vi "水样测试.vi"(11 "数据标记表":string(combo)="N") -> ()   [LabVIEW 2016, in "斯坦道多参数.lvlib"]
panel:
  out "运行状态":u16(ring) items=["空闲", "水样测试", "标样核查"]
  out "多参数运行日志":string
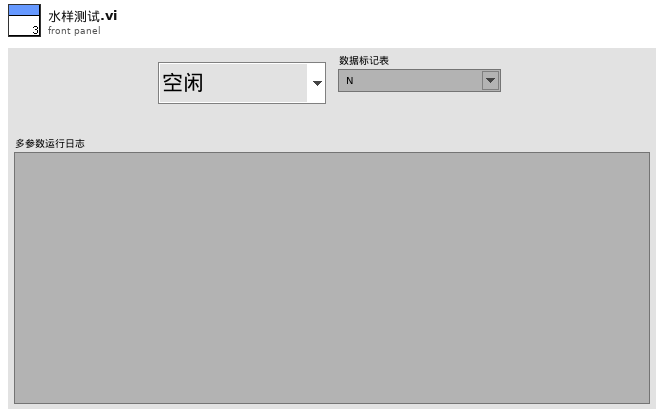
[diagram p1: front panel]
types:
  T1 = typedef "集成多参数单参数字段定义.ctl" = cluster{"时间":timestamp, "测量模式":string, "数据类型":string, "检测值":sgl, "单位":string, "数据标识":string, "标样参考值":sgl, "因子编码":string, "LastTime":timestamp}
  T2 = cluster{"水温":bool, "pH":bool, "DO":bool, "DOper":bool, "电导率":bool, "ORP":bool, "浊度":bool, "叶绿素a":bool, "藻密度":bool, "COD":bool, "DO2":bool, "DOper":bool, "氯化物":bool, "氨氮":bool, "水中油":bool}
  T3 = cluster{"ph":bool, "DO":bool, "Cond":bool, "Turb":bool, "叶绿素a":bool, "藻密度":bool, "ORP":bool, "cod":bool, "DO2":bool, "氯化物":bool, "氨氮":bool, "水中油":bool}
  T4 = cluster{"温度测量值":sgl, "测量值":sgl, "温度偏移修正值":sgl, "信号值":sgl, "数据标识":string}
  T5 = cluster{"温度测量值":sgl, "DO%":sgl, "DOmg/L":sgl, "温度偏移修正值":sgl, "数据标识mg/L":string, "数据标识%":string}
  T6 = cluster{"CH":u16, "监测值":dbl, "信号值":sgl, "数据标识":string}
  T7 = cluster{"水样数据时间":timestamp, "水温":dbl, "pH":dbl, "DO":dbl, "DOper":dbl, "电导率":dbl, "ORP":dbl, "浊度":dbl, "叶绿素a":dbl, "藻密度":dbl, "COD":dbl, "DO2":dbl, "DO2per":dbl, "氯化物":dbl, "氨氮":dbl, "水中油":dbl}
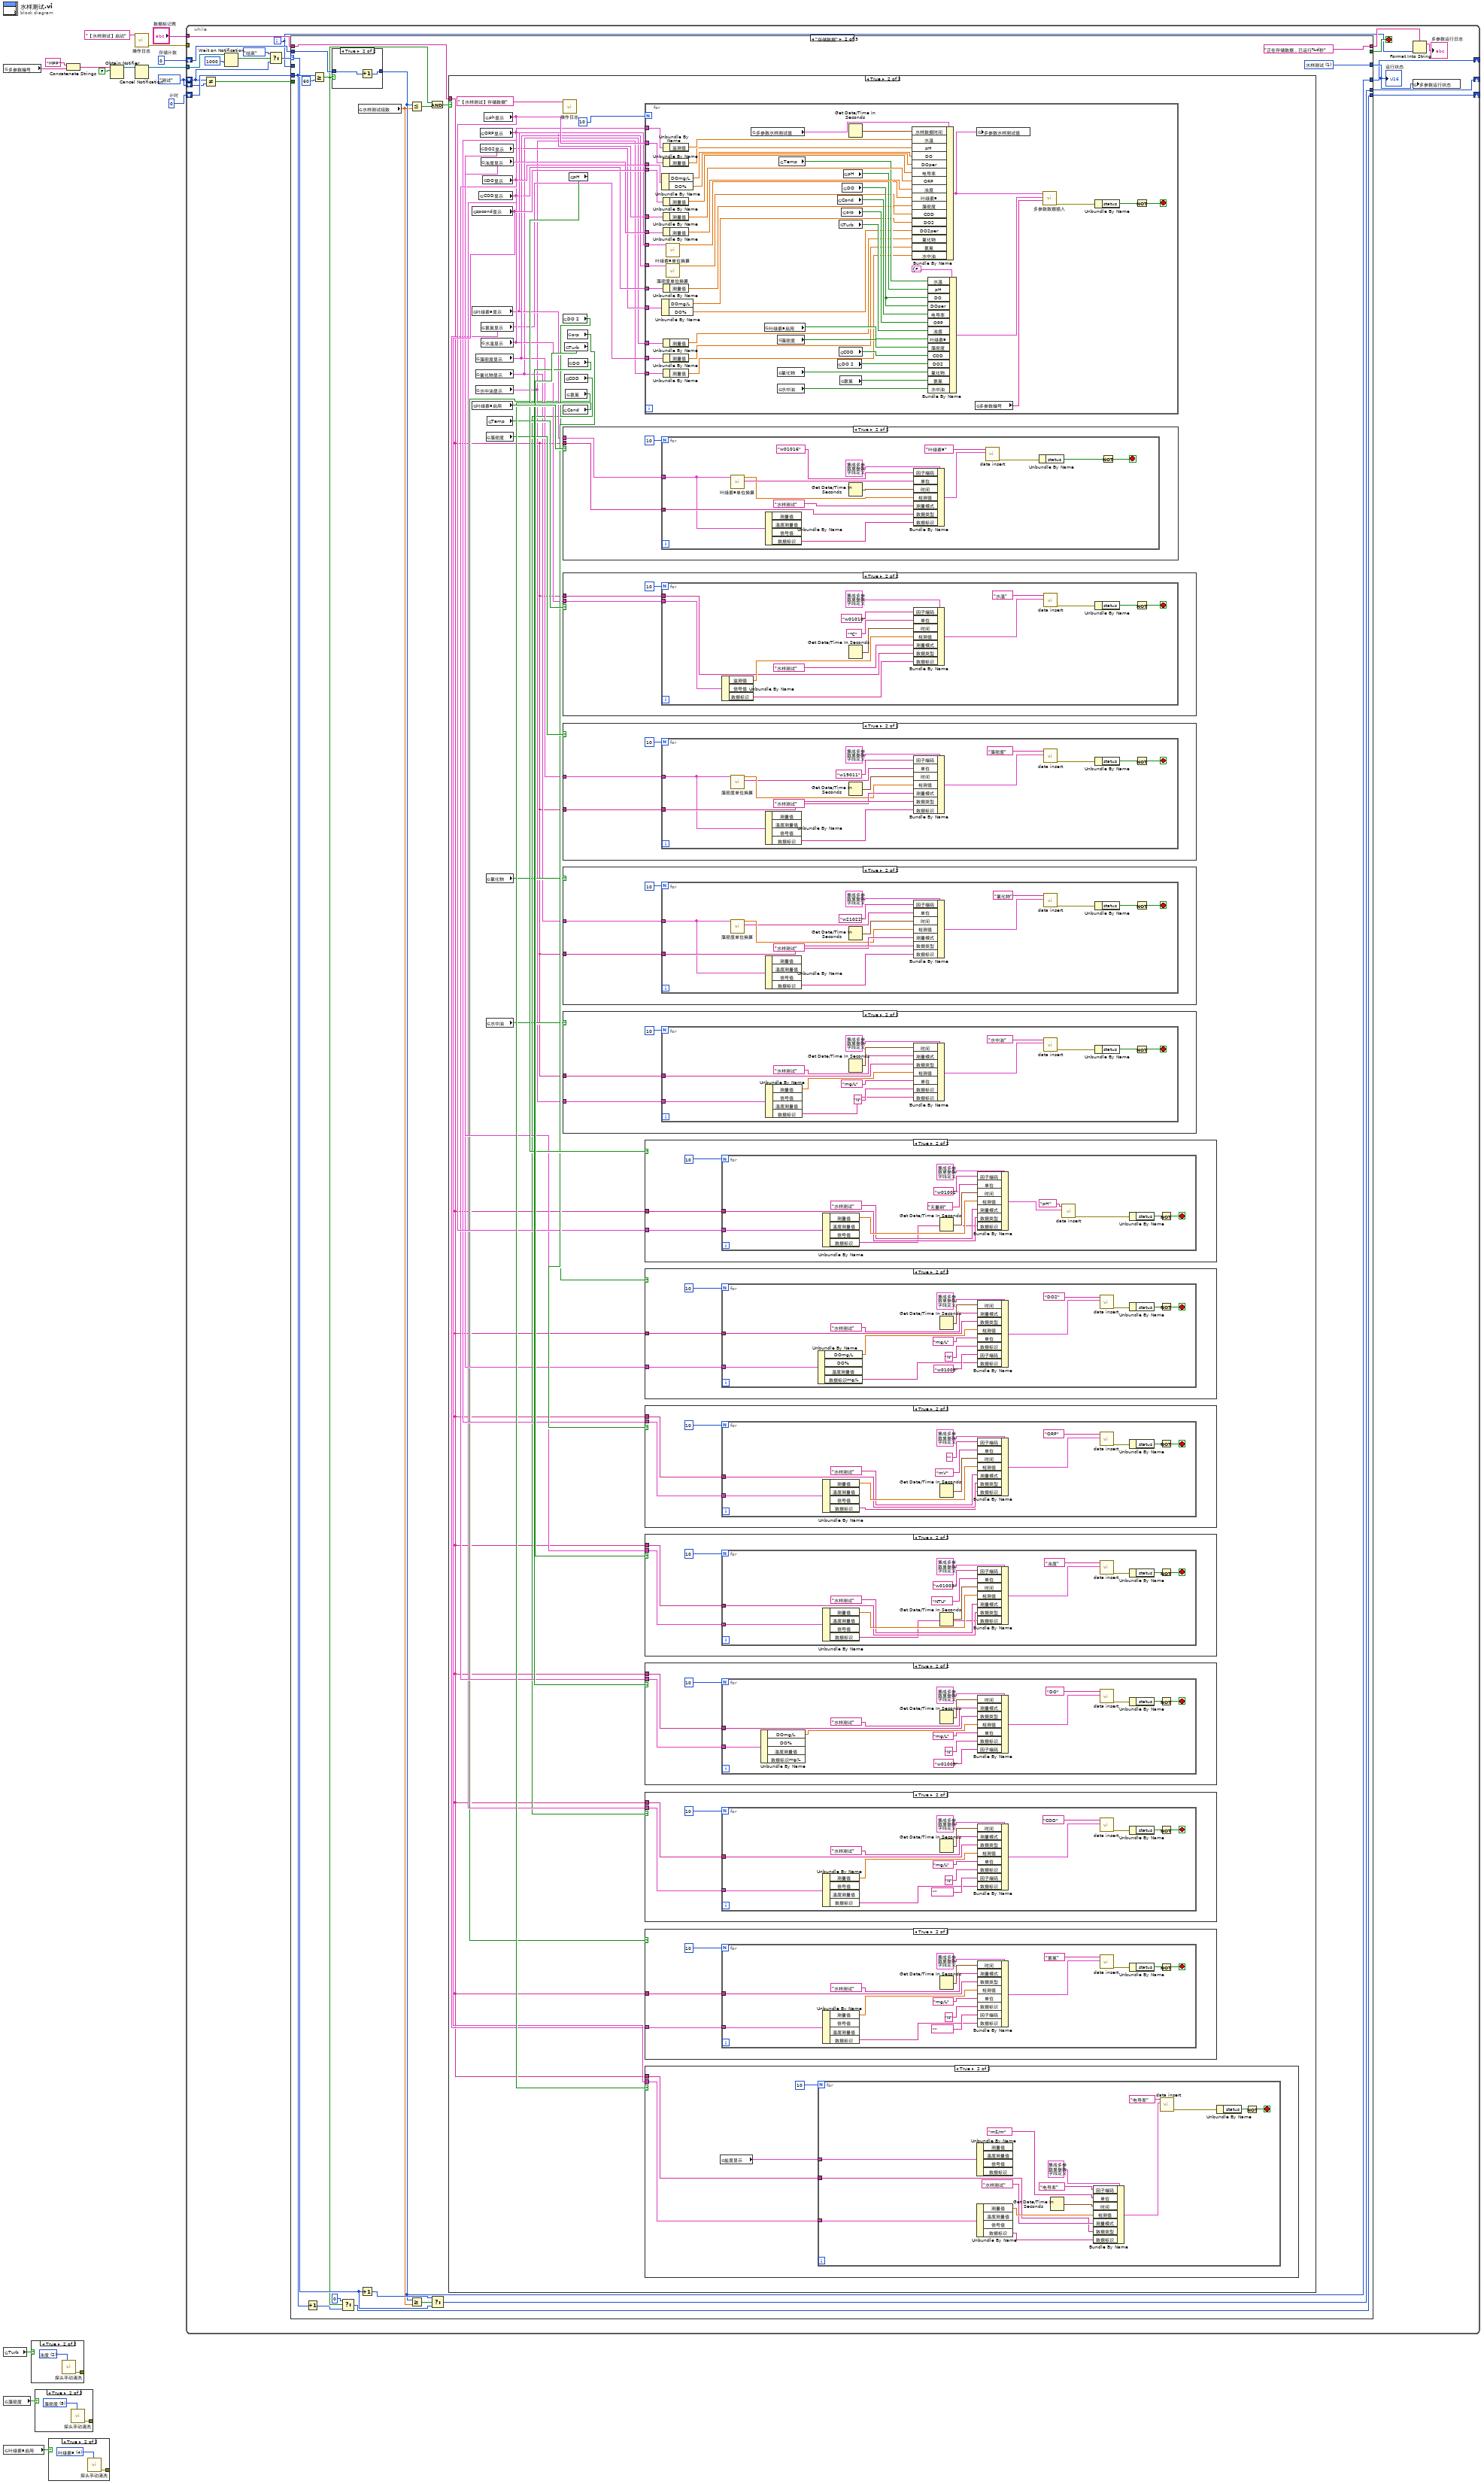
[diagram p0: block diagram]
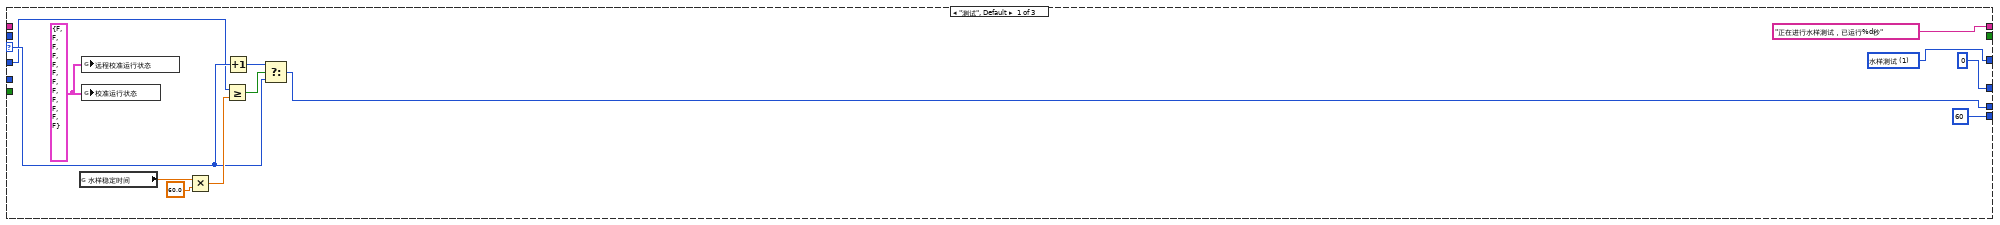
[diagram p5: hidden frame]
diagram:
  w7 = 0  # 存储计数
  w8 = 0  # 计时
  w3 = enum16{"测试", "存储数据", "结束"}."测试" ("枚举")
  n1 = global read "多参数全局变量.vi" "多参数编号"() -> (w9:string)
  n2 = global read "断电保存变量.vi" "Turb"() -> (w6:bool)
  n3 = global read "断电保存变量.vi" "藻密度"() -> (w4:bool)
  n4 = global read "断电保存变量.vi" "叶绿素a启用"() -> (w5:bool)
  n5 = case shown="True" w6 {
    tunnel: [_ w16] -> _
    frame False {
    }
    frame True {
      w17 = u16 2 items=["pH", "DO", "浊度", "电导率", "叶绿素a", "藻密度", "ORP", "DO2"] ("校准参数")
      n6 = call "探头手动清洗.vi"("校准参数"=w17) -> ("error out"=w16:errorcluster)  [unwired: 10 in]
    }
  }
  n7 = case shown="True" w4 {
    tunnel: [_ w18] -> _
    frame False {
    }
    frame True {
      w19 = u16 5 items=["pH", "DO", "浊度", "电导率", "叶绿素a", "藻密度", "ORP", "DO2"] ("校准参数")
      n8 = call "探头手动清洗.vi"("校准参数"=w19) -> ("error out"=w18:errorcluster)  [unwired: 10 in]
    }
  }
  n9 = case shown="True" w5 {
    tunnel: [_ w20] -> _
    frame False {
    }
    frame True {
      w21 = u16 4 items=["pH", "DO", "浊度", "电导率", "叶绿素a", "藻密度", "ORP", "DO2"] ("校准参数")
      n10 = call "探头手动清洗.vi"("校准参数"=w21) -> ("error out"=w20:errorcluster)  [unwired: 10 in]
    }
  }
  n11 = Concatenate Strings("MPP" ("名称（未命名）"), w9) -> (w10:string)
  n12 = Obtain Notifier(name (unnamed)=w10, notification data type=FALSE) -> (notifier out=w13:refnum<notifier>)  [unwired: 2 in, 2 out]
  n13 = call "操作日志.vi"("日志信息"="【水样测试】启动") -> ("error out"=w1:errorcluster)  [unwired: 10 in]
  n14 = Cancel Notification(0:w13) -> (8:w12:refnum<notifier>)  [unwired: 1 in, 2 out]
  n15 = while {
    shift-right: [w26] -> _
    shift-left: w3 -> [w24]
    tunnel: w12 -> [w37]
    tunnel: "数据标记表" -> [w32]
    shift-right: [w28] -> _
    shift-left: w8 -> [w30]
    shift-right: [w27] -> _
    shift-left: w7 -> [w29]
    shift-left: w3 -> [w23]
    tunnel: w1 -> [_]
    i -> [w25]
    stop <- w40 stop-if-true
    n16 = Not Equal?(x=w24, y=w23) -> (x != y?=w22:bool)
    n17 = Wait on Notification(notifier=w37, timeout in ms (-1)=1000 ("超时毫秒(-1)")) -> (notification=w35:bool)  [unwired: 2 in, 3 out]
    n18 = Select(t=enum16{"测试", "存储数据", "结束"}."结束" ("枚举"), s=w35, f=w24) -> (s? t:f=w33:enum16{"测试", "存储数据", "结束"})
    n19 = case shown="\"存储数据\"" w33 {
      selector: w33 -> [w47 w61 _]
      tunnel: [_ _ TRUE] -> w40
      tunnel: ["正在进行水样测试，已运行%d秒" ("格式字符串") "正在存储数据，已运行%d秒" ("格式字符串") "测试停止，累计运行%d秒" ("格式字符串")] -> w39
      tunnel: [w52 w66 w384] -> w31
      tunnel: w32 -> [_ w71 _]
      tunnel: w30 -> [_ w69 _]
      tunnel: w29 -> [_ w70 _]
      tunnel: [60 w54 0] -> w28
      tunnel: [0 w60 0] -> w27
      tunnel: [w45 w64 enum16{"测试", "存储数据", "结束"}."结束" ("枚举")] -> w26
      tunnel: w25 -> [w42 _ _]
      tunnel: w22 -> [_ _ w380]
      frame "测试", Default {
        w41 = T3 {"ph"=FALSE, "DO"=FALSE, "Cond"=FALSE, "Turb"=FALSE, "叶绿素a"=FALSE, "藻密度"=FALSE, "ORP"=FALSE, "cod"=FALSE, "DO2"=FALSE, "氯化物"=FALSE, "氨氮"=FALSE, "水中油"=FALSE} ("远程校准运行状态")
        w52 = u16 1 items=["空闲", "水样测试", "标样核查"] ("多参数运行状态")
        n20 = global read "断电保存变量.vi" "水样稳定时间"() -> (w51:dbl)
        n21 = global write "多参数全局变量.vi" "远程校准运行状态"(w41) -> ()
        n22 = global write "多参数全局变量.vi" "校准运行状态"(w41) -> ()
        n23 = Multiply(x=w51, y=60.0) -> (x*y=w49:dbl)
        n24 = Greater Or Equal?(x=w42, y=w49) -> (x >= y?=w48:bool)
        n25 = Increment(x=w47) -> (x+1=w46:enum16{"测试", "存储数据", "结束"})
        n26 = Select(t=w46, s=w48, f=w47) -> (s? t:f=w45:enum16{"测试", "存储数据", "结束"})
      }
      frame "存储数据" {
        w66 = u16 1 items=["空闲", "水样测试", "标样核查"] ("多参数运行状态")
        n27 = Increment(x=w69) -> (x+1=w56:i32)
        n28 = Greater Or Equal?(x=w69, y=60) -> (x >= y?=w57:bool)
        n29 = case shown="True" w57 {
          tunnel: w70 -> [w72 w74]
          tunnel: [w72 w73] -> w60
          frame False {
          }
          frame True {
            n30 = Increment(x=w74) -> (x+1=w73:i32)
          }
        }
        n31 = Select(t=0, s=w57, f=w56) -> (s? t:f=w54:i32)
        n32 = global read "断电保存变量.vi" "水样测试组数"() -> (w59:dbl)
        n33 = Increment(x=w61) -> (x+1=w62:enum16{"测试", "存储数据", "结束"})
        n34 = Less Or Equal?(x=w60, y=w59) -> (x <= y?=w65:bool)
        n35 = Greater Or Equal?(x=w60, y=w59) -> (x >= y?=w58:bool)
        n36 = And(x=w57, y=w65) -> (x .and. y?=w63:bool)
        n37 = Select(t=w62, s=w58, f=w61) -> (s? t:f=w64:enum16{"测试", "存储数据", "结束"})
        n38 = case shown="True" w63 {
          tunnel: w71 -> [_ w76]
          frame False {
          }
          frame True {
            n39 = global read "多参数全局变量.vi" "spcond显示"() -> (w94:T4)
            n40 = global read "多参数全局变量.vi" "叶绿素a显示"() -> (w88:T4)
            n41 = global read "断电保存变量.vi" "叶绿素a启用"() -> (w103:bool)
            n42 = global read "多参数全局变量.vi" "藻密度显示"() -> (w90:T4)
            n43 = global read "多参数全局变量.vi" "氯化物显示"() -> (w80:T4)
            n44 = global read "多参数全局变量.vi" "水中油显示"() -> (w75:T4)
            n45 = global read "多参数全局变量.vi" "COD显示"() -> (w85:T4)
            n46 = global read "多参数全局变量.vi" "ORP显示"() -> (w87:T4)
            n47 = global read "多参数全局变量.vi" "DO2显示"() -> (w82:T5)
            n48 = global read "多参数全局变量.vi" "浊度显示"() -> (w92:T4)
            n49 = global read "多参数全局变量.vi" "氨氮显示"() -> (w78:T4)
            n50 = global read "多参数全局变量.vi" "水温显示"() -> (w89:T6)
            n51 = global read "多参数全局变量.vi" "DO显示"() -> (w91:T5)
            n52 = global read "多参数全局变量.vi" "ph显示"() -> (w93:T4)
            n53 = global read "断电保存变量.vi" "藻密度"() -> (w97:bool)
            n54 = global read "断电保存变量.vi" "氯化物"() -> (w81:bool)
            n55 = global read "断电保存变量.vi" "水中油"() -> (w77:bool)
            n56 = global read "断电保存变量.vi" "Temp"() -> (w98:bool)
            n57 = call "操作日志.vi"("日志信息"="【水样测试】存储数据") -> ()  [unwired: 10 in, 1 out]
            n58 = global read "断电保存变量.vi" "DO 2"() -> (w83:bool)
            n59 = global read "断电保存变量.vi" "Cond"() -> (w101:bool)
            n60 = case shown="True" w103 {
              tunnel: w76 -> [_ w278]
              tunnel: w88 -> [_ w276]
              frame False {
              }
              frame True {
                n61 = for {
                  N: 10 -> [_]
                  tunnel: w278 -> [w284]
                  tunnel: w276 -> [w281]
                  stop <- w287 stop-if-true
                  n62 = call "叶绿素a单位换算.vi"("叶绿素a显示"=w281) -> ("检测值1.单位"=w280:string, "测量值"=w279:sgl)  [unwired: 8 in, 1 out]
                  n63 = Unbundle By Name(w281) -> ("数据标识"=w283:string)  [unwired: 3 out]
                  n64 = Get Date/Time In Seconds() -> (seconds since 1Jan1904=w286:timestamp)
                  n65 = Bundle By Name(cluster=T1 {"时间"=timestamp(0 s since 1904-01-01), "测量模式"="水样测试", "数据类型"="N", "检测值"=0.0, "单位"="mg/L", "数据标识"="N", "标样参考值"=0.0, "因子编码"="", "LastTime"=timestamp(0 s since 1904-01-01)} ("data"), "因子编码"="w01016", "单位"=w280, "时间"=w286, "检测值"=w279, "测量模式"="水样测试", "数据类型"=w284, "数据标识"=w283) -> (w291:T1)
                  n66 = call "data insert.vi"("data"=w291, "table in"="叶绿素a" ("table输入")) -> ("error out"=w289:errorcluster)  [unwired: 9 in]
                  n67 = Unbundle By Name(w289) -> ("status"=w288:bool)
                  n68 = Not(x=w288) -> (.not. x?=w287:bool)
                }
              }
            }
            n69 = case shown="True" w98 {
              tunnel: w76 -> [_ w365]
              tunnel: w89 -> [_ w363]
              frame False {
              }
              frame True {
                n70 = for {
                  N: 10 -> [_]
                  tunnel: w365 -> [w369]
                  tunnel: w363 -> [w368]
                  stop <- w372 stop-if-true
                  n71 = Unbundle By Name(w368) -> ("监测值"=w375:dbl, "数据标识"=w367:string)  [unwired: 1 out]
                  n72 = Get Date/Time In Seconds() -> (seconds since 1Jan1904=w371:timestamp)
                  n73 = Bundle By Name(cluster=T1 {"时间"=timestamp(0 s since 1904-01-01), "测量模式"="水样测试", "数据类型"="N", "检测值"=0.0, "单位"="mg/L", "数据标识"="N", "标样参考值"=0.0, "因子编码"="", "LastTime"=timestamp(0 s since 1904-01-01)} ("data"), "因子编码"="w01010", "单位"="℃", "时间"=w371, "检测值"=w375, "测量模式"="水样测试", "数据类型"=w369, "数据标识"=w367) -> (w378:T1)
                  n74 = call "data insert.vi"("data"=w378, "table in"="水温" ("table输入")) -> ("error out"=w374:errorcluster)  [unwired: 9 in]
                  n75 = Unbundle By Name(w374) -> ("status"=w373:bool)
                  n76 = Not(x=w373) -> (.not. x?=w372:bool)
                }
              }
            }
            n77 = case shown="True" w97 {
              tunnel: w76 -> [_ w261]
              tunnel: w90 -> [_ w259]
              frame False {
              }
              frame True {
                n78 = for {
                  N: 10 -> [_]
                  tunnel: w261 -> [w268]
                  tunnel: w259 -> [w264]
                  stop <- w269 stop-if-true
                  n79 = call "藻密度单位换算.vi"("藻密度显示"=w264) -> ("检测值1.单位"=w262:string, "测量值"=w263:sgl)  [unwired: 8 in, 1 out]
                  n80 = Unbundle By Name(w264) -> ("数据标识"=w266:string)  [unwired: 3 out]
                  n81 = Get Date/Time In Seconds() -> (seconds since 1Jan1904=w270:timestamp)
                  n82 = Bundle By Name(cluster=T1 {"时间"=timestamp(0 s since 1904-01-01), "测量模式"="水样测试", "数据类型"="N", "检测值"=0.0, "单位"="mg/L", "数据标识"="N", "标样参考值"=0.0, "因子编码"="", "LastTime"=timestamp(0 s since 1904-01-01)} ("data"), "因子编码"="w19011", "单位"=w262, "时间"=w270, "检测值"=w263, "测量模式"="水样测试", "数据类型"=w268, "数据标识"=w266) -> (w271:T1)
                  n83 = call "data insert.vi"("data"=w271, "table in"="藻密度" ("table输入")) -> ("error out"=w273:errorcluster)  [unwired: 9 in]
                  n84 = Unbundle By Name(w273) -> ("status"=w272:bool)
                  n85 = Not(x=w272) -> (.not. x?=w269:bool)
                }
              }
            }
            n86 = case shown="True" w81 {
              tunnel: w76 -> [_ w141]
              tunnel: w80 -> [_ w139]
              frame False {
              }
              frame True {
                n87 = for {
                  N: 10 -> [_]
                  tunnel: w141 -> [w150]
                  tunnel: w139 -> [w146]
                  stop <- w151 stop-if-true
                  n88 = call "藻密度单位换算.vi"("藻密度显示"=w146) -> ("检测值1.单位"=w144:string, "测量值"=w145:sgl)  [unwired: 8 in, 1 out]
                  n89 = Unbundle By Name(w146) -> ("数据标识"=w148:string)  [unwired: 3 out]
                  n90 = Get Date/Time In Seconds() -> (seconds since 1Jan1904=w152:timestamp)
                  n91 = Bundle By Name(cluster=T1 {"时间"=timestamp(0 s since 1904-01-01), "测量模式"="水样测试", "数据类型"="N", "检测值"=0.0, "单位"="mg/L", "数据标识"="N", "标样参考值"=0.0, "因子编码"="", "LastTime"=timestamp(0 s since 1904-01-01)} ("data"), "因子编码"="w21022", "单位"=w144, "时间"=w152, "检测值"=w145, "测量模式"="水样测试", "数据类型"=w150, "数据标识"=w148) -> (w153:T1)
                  n92 = call "data insert.vi"("data"=w153, "table in"="氯化物") -> ("error out"=w155:errorcluster)  [unwired: 9 in]
                  n93 = Unbundle By Name(w155) -> ("status"=w154:bool)
                  n94 = Not(x=w154) -> (.not. x?=w151:bool)
                }
              }
            }
            n95 = case shown="True" w77 {
              tunnel: w76 -> [_ w106]
              tunnel: w75 -> [_ w104]
              frame False {
              }
              frame True {
                n96 = for {
                  N: 10 -> [_]
                  tunnel: w106 -> [w117]
                  tunnel: w104 -> [w110]
                  stop <- w120 stop-if-true
                  n97 = Unbundle By Name(w110) -> ("测量值"=w109:sgl, "数据标识"=w108:string)  [unwired: 2 out]
                  n98 = Get Date/Time In Seconds() -> (seconds since 1Jan1904=w119:timestamp)
                  n99 = Bundle By Name(cluster=T1 {"时间"=timestamp(0 s since 1904-01-01), "测量模式"="水样测试", "数据类型"="N", "检测值"=0.0, "单位"="mg/L", "数据标识"="N", "标样参考值"=0.0, "因子编码"="", "LastTime"=timestamp(0 s since 1904-01-01)} ("data"), "时间"=w119, "测量模式"="水样测试", "数据类型"=w117, "检测值"=w109, "单位"="mg/L", "数据标识"="N" ("水样数据标识"), "数据标识"=w108) -> (w112:T1)
                  n100 = call "data insert.vi"("data"=w112, "table in"="水中油") -> ("error out"=w113:errorcluster)  [unwired: 9 in]
                  n101 = Unbundle By Name(w113) -> ("status"=w114:bool)
                  n102 = Not(x=w114) -> (.not. x?=w120:bool)
                }
              }
            }
            n103 = global read "断电保存变量.vi" "Turb"() -> (w102:bool)
            n104 = global read "断电保存变量.vi" "COD"() -> (w84:bool)
            n105 = global read "断电保存变量.vi" "氨氮"() -> (w79:bool)
            n106 = global read "断电保存变量.vi" "orp"() -> (w96:bool)
            n107 = global read "断电保存变量.vi" "DO"() -> (w100:bool)
            n108 = global read "断电保存变量.vi" "pH"() -> (w99:bool)
            n109 = for {
              N: 10 -> [_]
              tunnel: w89 -> [w221]
              tunnel: w93 -> [w220]
              tunnel: w91 -> [w219]
              tunnel: w94 -> [w218]
              tunnel: w87 -> [w217]
              tunnel: w92 -> [w216]
              tunnel: w88 -> [w206]
              tunnel: w90 -> [w208]
              tunnel: w85 -> [w214]
              tunnel: w82 -> [w211]
              tunnel: w80 -> [w202]
              tunnel: w78 -> [w200]
              tunnel: w75 -> [w193]
              stop <- w223 stop-if-true
              n110 = Unbundle By Name(w219) -> ("DOmg/L"=w238:sgl, "DO%"=w237:sgl)
              n111 = Unbundle By Name(w211) -> ("DOmg/L"=w210:sgl, "DO%"=w209:sgl)
              n112 = Unbundle By Name(w221) -> ("监测值"=w240:dbl)
              n113 = Unbundle By Name(w220) -> ("测量值"=w239:sgl)
              n114 = Unbundle By Name(w218) -> ("测量值"=w236:sgl)
              n115 = Unbundle By Name(w217) -> ("测量值"=w235:sgl)
              n116 = Unbundle By Name(w216) -> ("测量值"=w234:sgl)
              n117 = Unbundle By Name(w214) -> ("测量值"=w213:sgl)
              n118 = Unbundle By Name(w202) -> ("测量值"=w201:sgl)
              n119 = Unbundle By Name(w200) -> ("测量值"=w199:sgl)
              n120 = Unbundle By Name(w193) -> ("测量值"=w192:sgl)
              n121 = call "叶绿素a单位换算.vi"("叶绿素a显示"=w206) -> ("测量值"=w205:sgl)  [unwired: 8 in, 2 out]
              n122 = call "藻密度单位换算.vi"("藻密度显示"=w208) -> ("测量值"=w207:sgl)  [unwired: 8 in, 2 out]
              n123 = global read "多参数全局变量.vi" "多参数水样测试值"() -> (w197:T7)
              n124 = global read "断电保存变量.vi" "叶绿素a启用"() -> (w227:bool)
              n125 = global read "断电保存变量.vi" "藻密度"() -> (w230:bool)
              n126 = global read "断电保存变量.vi" "氯化物"() -> (w203:bool)
              n127 = global read "断电保存变量.vi" "水中油"() -> (w194:bool)
              n128 = global read "断电保存变量.vi" "Temp"() -> (w229:bool)
              n129 = global read "断电保存变量.vi" "Cond"() -> (w232:bool)
              n130 = global read "断电保存变量.vi" "DO 2"() -> (w212:bool)
              n131 = global read "断电保存变量.vi" "Turb"() -> (w231:bool)
              n132 = global read "断电保存变量.vi" "COD"() -> (w215:bool)
              n133 = global read "断电保存变量.vi" "氨氮"() -> (w198:bool)
              n134 = global read "断电保存变量.vi" "orp"() -> (w228:bool)
              n135 = global read "断电保存变量.vi" "DO"() -> (w226:bool)
              n136 = global read "断电保存变量.vi" "pH"() -> (w233:bool)
              n137 = Get Date/Time In Seconds() -> (seconds since 1Jan1904=w241:timestamp)
              n138 = Bundle By Name(cluster=w197, "水样数据时间"=w241, "水温"=w240, "pH"=w239, "DO"=w238, "DOper"=w237, "电导率"=w236, "ORP"=w235, "浊度"=w234, "叶绿素a"=w205, "藻密度"=w207, "COD"=w213, "DO2"=w210, "DO2per"=w209, "氯化物"=w201, "氨氮"=w199, "水中油"=w192) -> (w204:T7)
              n139 = Bundle By Name(cluster=T2 {"水温"=FALSE, "pH"=FALSE, "DO"=FALSE, "DOper"=FALSE, "电导率"=FALSE, "ORP"=FALSE, "浊度"=FALSE, "叶绿素a"=FALSE, "藻密度"=FALSE, "COD"=FALSE, "DO2"=FALSE, "DOper"=FALSE, "氯化物"=FALSE, "氨氮"=FALSE, "水中油"=FALSE} ("columns enable"), "水温"=w229, "pH"=w233, "DO"=w226, "DOper"=w226, "电导率"=w232, "ORP"=w228, "浊度"=w231, "叶绿素a"=w227, "藻密度"=w230, "COD"=w215, "DO2"=w212, "氯化物"=w203, "氨氮"=w198, "水中油"=w194) -> (w195:T2)
              n140 = global read "多参数全局变量.vi" "多参数编号"() -> (w222:string)
              n141 = global write "多参数全局变量.vi" "多参数水样测试值"(w204) -> ()
              n142 = call "多参数数据插入.vi"("编号"=w222, "columns enable"=w195, "data in"=w204) -> ("error out"=w225:errorcluster)  [unwired: 8 in]
              n143 = Unbundle By Name(w225) -> ("status"=w224:bool)
              n144 = Not(x=w224) -> (.not. x?=w223:bool)
            }
            n145 = case shown="True" w99 {
              tunnel: w76 -> [_ w348]
              tunnel: w93 -> [_ w346]
              frame False {
              }
              frame True {
                n146 = for {
                  N: 10 -> [_]
                  tunnel: w348 -> [w352]
                  tunnel: w346 -> [w351]
                  stop <- w355 stop-if-true
                  n147 = Unbundle By Name(w351) -> ("测量值"=w358:sgl, "数据标识"=w350:string)  [unwired: 2 out]
                  n148 = Get Date/Time In Seconds() -> (seconds since 1Jan1904=w354:timestamp)
                  n149 = Bundle By Name(cluster=T1 {"时间"=timestamp(0 s since 1904-01-01), "测量模式"="水样测试", "数据类型"="N", "检测值"=0.0, "单位"="mg/L", "数据标识"="N", "标样参考值"=0.0, "因子编码"="", "LastTime"=timestamp(0 s since 1904-01-01)} ("data"), "因子编码"="w01001", "单位"="无量纲", "时间"=w354, "检测值"=w358, "测量模式"="水样测试", "数据类型"=w352, "数据标识"=w350) -> (w362:T1)
                  n150 = call "data insert.vi"("data"=w362, "table in"="pH" ("table输入")) -> ("error out"=w357:errorcluster)  [unwired: 9 in]
                  n151 = Unbundle By Name(w357) -> ("status"=w356:bool)
                  n152 = Not(x=w356) -> (.not. x?=w355:bool)
                }
              }
            }
            n153 = case shown="True" w83 {
              tunnel: w76 -> [_ w158]
              tunnel: w82 -> [_ w156]
              frame False {
              }
              frame True {
                n154 = for {
                  N: 10 -> [_]
                  tunnel: w158 -> [w170]
                  tunnel: w156 -> [w162]
                  stop <- w173 stop-if-true
                  n155 = Unbundle By Name(w162) -> ("DOmg/L"=w169:sgl, "数据标识mg/L"=w161:string)  [unwired: 2 out]
                  n156 = Get Date/Time In Seconds() -> (seconds since 1Jan1904=w172:timestamp)
                  n157 = Bundle By Name(cluster=T1 {"时间"=timestamp(0 s since 1904-01-01), "测量模式"="水样测试", "数据类型"="N", "检测值"=0.0, "单位"="mg/L", "数据标识"="N", "标样参考值"=0.0, "因子编码"="", "LastTime"=timestamp(0 s since 1904-01-01)} ("data"), "时间"=w172, "测量模式"="水样测试", "数据类型"=w170, "检测值"=w169, "单位"="mg/L", "数据标识"="N" ("水样数据标识"), "因子编码"="w01009", "数据标识"=w161) -> (w163:T1)
                  n158 = call "data insert.vi"("data"=w163, "table in"="DO2") -> ("error out"=w165:errorcluster)  [unwired: 9 in]
                  n159 = Unbundle By Name(w165) -> ("status"=w166:bool)
                  n160 = Not(x=w166) -> (.not. x?=w173:bool)
                }
              }
            }
            n161 = case shown="True" w96 {
              tunnel: w76 -> [_ w244]
              tunnel: w87 -> [_ w242]
              frame False {
              }
              frame True {
                n162 = for {
                  N: 10 -> [_]
                  tunnel: w244 -> [w250]
                  tunnel: w242 -> [w248]
                  stop <- w252 stop-if-true
                  n163 = Unbundle By Name(w248) -> ("测量值"=w258:sgl, "数据标识"=w247:string)  [unwired: 2 out]
                  n164 = Get Date/Time In Seconds() -> (seconds since 1Jan1904=w251:timestamp)
                  n165 = Bundle By Name(cluster=T1 {"时间"=timestamp(0 s since 1904-01-01), "测量模式"="水样测试", "数据类型"="N", "检测值"=0.0, "单位"="mg/L", "数据标识"="N", "标样参考值"=0.0, "因子编码"="", "LastTime"=timestamp(0 s since 1904-01-01)} ("data"), "因子编码"="", "单位"="mV", "时间"=w251, "检测值"=w258, "测量模式"="水样测试", "数据类型"=w250, "数据标识"=w247) -> (w245:T1)
                  n166 = call "data insert.vi"("data"=w245, "table in"="ORP" ("table输入")) -> ("error out"=w255:errorcluster)  [unwired: 9 in]
                  n167 = Unbundle By Name(w255) -> ("status"=w254:bool)
                  n168 = Not(x=w254) -> (.not. x?=w252:bool)
                }
              }
            }
            n169 = case shown="True" w102 {
              tunnel: w76 -> [_ w295]
              tunnel: w92 -> [_ w293]
              frame False {
              }
              frame True {
                n170 = for {
                  N: 10 -> [_]
                  tunnel: w295 -> [w299]
                  tunnel: w293 -> [w298]
                  stop <- w302 stop-if-true
                  n171 = Unbundle By Name(w298) -> ("测量值"=w305:sgl, "数据标识"=w297:string)  [unwired: 2 out]
                  n172 = Get Date/Time In Seconds() -> (seconds since 1Jan1904=w301:timestamp)
                  n173 = Bundle By Name(cluster=T1 {"时间"=timestamp(0 s since 1904-01-01), "测量模式"="水样测试", "数据类型"="N", "检测值"=0.0, "单位"="mg/L", "数据标识"="N", "标样参考值"=0.0, "因子编码"="", "LastTime"=timestamp(0 s since 1904-01-01)} ("data"), "因子编码"="w01003", "单位"="NTU", "时间"=w301, "检测值"=w305, "测量模式"="水样测试", "数据类型"=w299, "数据标识"=w297) -> (w308:T1)
                  n174 = call "data insert.vi"("data"=w308, "table in"="浊度" ("table输入")) -> ("error out"=w304:errorcluster)  [unwired: 9 in]
                  n175 = Unbundle By Name(w304) -> ("status"=w303:bool)
                  n176 = Not(x=w303) -> (.not. x?=w302:bool)
                }
              }
            }
            n177 = case shown="True" w100 {
              tunnel: w76 -> [_ w331]
              tunnel: w91 -> [_ w329]
              frame False {
              }
              frame True {
                n178 = for {
                  N: 10 -> [_]
                  tunnel: w331 -> [w341]
                  tunnel: w329 -> [w334]
                  stop <- w345 stop-if-true
                  n179 = Unbundle By Name(w334) -> ("DOmg/L"=w340:sgl)  [unwired: 3 out]
                  n180 = Get Date/Time In Seconds() -> (seconds since 1Jan1904=w343:timestamp)
                  n181 = Bundle By Name(cluster=T1 {"时间"=timestamp(0 s since 1904-01-01), "测量模式"="水样测试", "数据类型"="N", "检测值"=0.0, "单位"="mg/L", "数据标识"="N", "标样参考值"=0.0, "因子编码"="", "LastTime"=timestamp(0 s since 1904-01-01)} ("data"), "时间"=w343, "测量模式"="水样测试", "数据类型"=w341, "检测值"=w340, "单位"="mg/L", "数据标识"="N", "因子编码"="w01009") -> (w335:T1)
                  n182 = call "data insert.vi"("data"=w335, "table in"="DO") -> ("error out"=w337:errorcluster)  [unwired: 9 in]
                  n183 = Unbundle By Name(w337) -> ("status"=w338:bool)
                  n184 = Not(x=w338) -> (.not. x?=w345:bool)
                }
              }
            }
            n185 = case shown="True" w84 {
              tunnel: w76 -> [_ w176]
              tunnel: w85 -> [_ w174]
              frame False {
              }
              frame True {
                n186 = for {
                  N: 10 -> [_]
                  tunnel: w176 -> [w187]
                  tunnel: w174 -> [w179]
                  stop <- w191 stop-if-true
                  n187 = Unbundle By Name(w179) -> ("测量值"=w186:sgl, "数据标识"=w178:string)  [unwired: 2 out]
                  n188 = Get Date/Time In Seconds() -> (seconds since 1Jan1904=w189:timestamp)
                  n189 = Bundle By Name(cluster=T1 {"时间"=timestamp(0 s since 1904-01-01), "测量模式"="水样测试", "数据类型"="N", "检测值"=0.0, "单位"="mg/L", "数据标识"="N", "标样参考值"=0.0, "因子编码"="", "LastTime"=timestamp(0 s since 1904-01-01)} ("data"), "时间"=w189, "测量模式"="水样测试", "数据类型"=w187, "检测值"=w186, "单位"="mg/L", "数据标识"="N" ("水样数据标识"), "因子编码"="", "数据标识"=w178) -> (w180:T1)
                  n190 = call "data insert.vi"("data"=w180, "table in"="COD") -> ("error out"=w182:errorcluster)  [unwired: 9 in]
                  n191 = Unbundle By Name(w182) -> ("status"=w183:bool)
                  n192 = Not(x=w183) -> (.not. x?=w191:bool)
                }
              }
            }
            n193 = case shown="True" w79 {
              tunnel: w76 -> [_ w123]
              tunnel: w78 -> [_ w121]
              frame False {
              }
              frame True {
                n194 = for {
                  N: 10 -> [_]
                  tunnel: w123 -> [w134]
                  tunnel: w121 -> [w126]
                  stop <- w138 stop-if-true
                  n195 = Unbundle By Name(w126) -> ("测量值"=w125:sgl, "数据标识"=w124:string)  [unwired: 2 out]
                  n196 = Get Date/Time In Seconds() -> (seconds since 1Jan1904=w136:timestamp)
                  n197 = Bundle By Name(cluster=T1 {"时间"=timestamp(0 s since 1904-01-01), "测量模式"="水样测试", "数据类型"="N", "检测值"=0.0, "单位"="mg/L", "数据标识"="N", "标样参考值"=0.0, "因子编码"="", "LastTime"=timestamp(0 s since 1904-01-01)} ("data"), "时间"=w136, "测量模式"="水样测试", "数据类型"=w134, "检测值"=w125, "单位"="mg/L", "数据标识"="N" ("水样数据标识"), "因子编码"="", "数据标识"=w124) -> (w128:T1)
                  n198 = call "data insert.vi"("data"=w128, "table in"="氨氮") -> ("error out"=w130:errorcluster)  [unwired: 9 in]
                  n199 = Unbundle By Name(w130) -> ("status"=w131:bool)
                  n200 = Not(x=w131) -> (.not. x?=w138:bool)
                }
              }
            }
            n201 = case shown="True" w101 {
              tunnel: w76 -> [_ w313]
              tunnel: w94 -> [_ w311]
              frame False {
              }
              frame True {
                n202 = global read "多参数全局变量.vi" "盐度显示"() -> (w310:T4)
                n203 = for {
                  N: 10 -> [_]
                  tunnel: w313 -> [w316]
                  tunnel: w311 -> [w319]
                  tunnel: w310 -> [w315]
                  stop <- w323 stop-if-true
                  n204 = Unbundle By Name(w315) -> ()  [unwired: 4 out]
                  n205 = Unbundle By Name(w319) -> ("测量值"=w326:sgl, "数据标识"=w318:string)  [unwired: 2 out]
                  n206 = Get Date/Time In Seconds() -> (seconds since 1Jan1904=w322:timestamp)
                  n207 = Bundle By Name(cluster=T1 {"时间"=timestamp(0 s since 1904-01-01), "测量模式"="水样测试", "数据类型"="N", "检测值"=0.0, "单位"="mg/L", "数据标识"="N", "标样参考值"=0.0, "因子编码"="", "LastTime"=timestamp(0 s since 1904-01-01)} ("data"), "因子编码"="电导率", "单位"="mS/m", "时间"=w322, "检测值"=w326, "测量模式"="水样测试", "数据类型"=w316, "数据标识"=w318) -> (w320:T1)
                  n208 = call "data insert.vi"("data"=w320, "table in"="电导率" ("table输入")) -> ("error out"=w314:errorcluster)  [unwired: 9 in]
                  n209 = Unbundle By Name(w314) -> ("status"=w325:bool)
                  n210 = Not(x=w325) -> (.not. x?=w323:bool)
                }
              }
            }
          }
        }
      }
      frame "结束" {
        w384 = u16 0 items=["空闲", "水样测试", "标样核查"] ("多参数运行状态")
        n211 = case shown="True" w380 {
          frame False {
          }
          frame True {
            n212 = call "操作日志.vi"("日志信息"="【水样测试】结束") -> ()  [unwired: 10 in, 1 out]
          }
        }
      }
    }
    "运行状态" <- w31
    n213 = Format Into String(format string=w39, w25) -> (resulting string=→"多参数运行日志":string)  [unwired: 2 in, 1 out]
    n214 = global write "多参数全局变量.vi" "多参数运行状态"(w31) -> ()
  }
